vi "dfd_Get Filter Freq Resp on Freq Pts.vi"(6 "fs [Hz]":dbl, 7 "freqs [Hz]":dbl[](array[numeric]), 8 "error in (no error)":errorcluster, 10 "coef source":enum16{"Original", "Current", "Quantized"}(ring), 11 "filter in":T1 {"mSRate_QSettings"."source" items=["Coef a/k"=0, "Coef b/v"=7, "Input"=1, "Output"=2, "Multiplicand"=3, "Product"=4, "Sum"=5, "Delay"=6, "Gain"=8]}) -> (0 "error out":errorcluster, 3 "freq response":cdb[](array[numeric]))   [LabVIEW 2017, in "NI_DigFilterLicensed.lvlib"]
uses:
  <vilib>/addons/Digital Filter Design/NI_DigFilterLicensed.lvlib
  <vilib>/addons/Digital Filter Design/_Objects.llb/DFD Filter Obj.ctl
  <vilib>/addons/Digital Filter Design/_Objects.llb/DFD Filter Coef.ctl
  <vilib>/addons/Digital Filter Design/_Objects.llb/DFD Filter Structure Type Selector.ctl
  <vilib>/addons/Digital Filter Design/_Objects.llb/dfd_Internal Quantization Settings.ctl
  <vilib>/addons/Digital Filter Design/_Objects.llb/dfd_Internal Quantization Srcs.ctl
  <vilib>/addons/Digital Filter Design/_Objects.llb/DFD Coef Norm Type.ctl
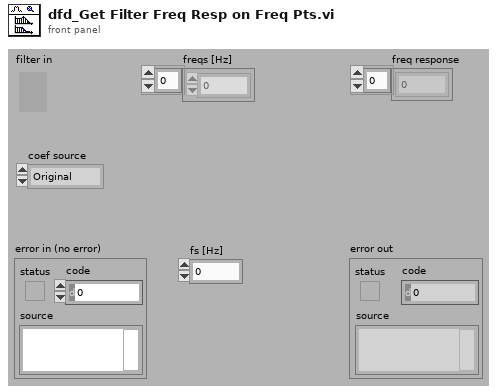
[diagram p1: front panel]
types:
  T1 = typedef "NI_DigFilterLicensed.lvlib/DFD Filter Obj.ctl" = cluster{"mSRate_Fs":dbl, "mSRate_Version":string, "mSRate_Comments":string, "mSRate_OrgCoef":T2, "mSRate_CurCoef":T2, "mSRate_Quantized?":bool, "mSRate_QCoef":T2, "mSRate_QSettings":T4[], "mSRate_Order":i32, "mSRate_Scaling":cluster{"mSRate_ScaleByPowerOf2?":bool, "mSRate_ScaleType":T6}}
  T2 = typedef "NI_DigFilterLicensed.lvlib/DFD Filter Coef.ctl" = cluster{"type":T3, "gain":dbl, "coef a (k)":dbl[], "coef b (v)":dbl[]}
  T3 = typedef "NI_DigFilterLicensed.lvlib/DFD Filter Structure Type Selector.ctl" = enum16{"Undefined", "FIR Direct Form", "FIR Direct Form Transposed", "FIR Symmetric", "FIR Antisymmetric", "IIR Direct Form I", "IIR Direct Form I Transposed", "IIR Direct Form II", "IIR Direct Form II Transposed", "IIR Cascaded Second Order Sections Form I", "IIR Cascaded Second Order Sections Form I Transposed", "IIR Cascaded Second Order Sections Form II", "IIR Cascaded Second Order Sections Form II Transposed", "Lattice Allpass (basic sections)", "Lattice Allpass (one multiplier sections)", "Lattice Allpass (normalized sections)", "Lattice AR (basic sections)", "Lattice AR (one multiplier sections)", "Lattice AR (normalized sections)", "Lattice MA (minimum phase)", "Lattice MA (maximum phase)", "Lattice ARMA (basic sections)", "Lattice ARMA (one multiplier sections)", "Lattice ARMA (normalized sections)"}
  T4 = typedef "NI_DigFilterLicensed.lvlib/dfd_Internal Quantization Settings.ctl" = cluster{"source":T5, "wl":i16, "iwl":i16, "overflow mode":enum16{"Saturation", "Wrap"}, "rounding mode":enum16{"Nearest", "Truncation"}, "signed?":bool}
  T5 = typedef "NI_DigFilterLicensed.lvlib/dfd_Internal Quantization Srcs.ctl" = u16
  T6 = typedef "NI_DigFilterLicensed.lvlib/DFD Coef Norm Type.ctl" = enum16{"No Norm", "Time Domain 1-Norm", "Time Domain 2-Norm", "Time Domain Inf-Norm"}
  T7 = typedef "NI_DigFilterLicensed.lvlib/DFD Filter Structure Id.ctl" = enum16{"Undefined", "FIR", "IIR Direct", "IIR SOS", "IIR Allpass", "IIR AR", "IIR ARMA"}
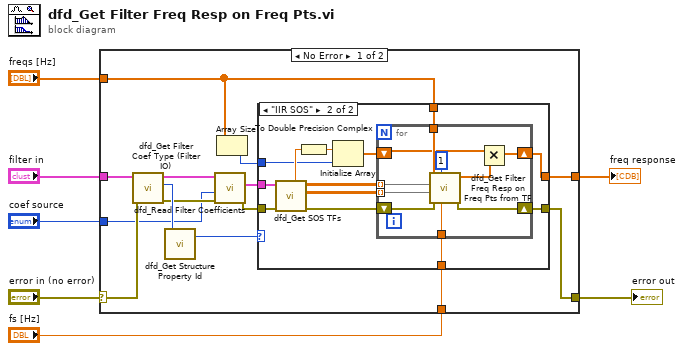
[diagram p0: block diagram]
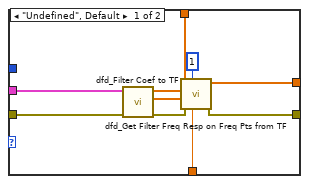
[diagram p2: hidden frame]
diagram:
  n1 = case shown="No Error" "error in (no error)" {
    selector: "error in (no error)" -> [w18 w55]
    tunnel: "coef source" -> [w14 _]
    tunnel: [w21 _] -> w6
    tunnel: "filter in" -> [w19 _]
    tunnel: "freqs [Hz]" -> [w10 _]
    tunnel: "fs [Hz]" -> [w20 _]
    tunnel: [w8 w55] -> w1
    frame No Error {
      n2 = call <vilib>:"dfd_Get Filter Coef Type (Filter IO).vi"("error in (no error)"=w18, "filter in"=w19) -> ("error out"=w15:errorcluster, "type"=w17:T3, "filter out"=w16:T1)  [unwired: 1 in, 6 out]
      n3 = call <vilib>:"dfd_Get Structure Property Id.vi"("structure type"=w17) -> ("filter structure id"=w13:T7)  [unwired: 1 out]
      n4 = call <vilib>:"dfd_Read Filter Coefficients.vi"("error in (no error)"=w15, "coef source"=w14, "filter in"=w16) -> ("error out"=w11:errorcluster, "filter coef"=w12:T2)  [unwired: 7 out]
      n5 = Array Size(array=w10) -> (size(s)=w9:i32)
      n6 = case shown="\"IIR SOS\"" w13 {
        tunnel: [w30 w37] -> w21
        tunnel: w10 -> [w26 w39]
        tunnel: w20 -> [w25 w38]
        tunnel: w12 -> [w24 w44]
        tunnel: w11 -> [w23 w43]
        tunnel: w9 -> [_ w34]
        tunnel: [w22 w32] -> w8
        frame "Undefined", Default {
          n7 = call <vilib>:"dfd_Filter Coef to TF.vi"("error out"=w23, "filter coef"=w24) -> ("error"=w29:errorcluster, "denominator"=w28:dbl[], "numerator"=w27:dbl[])  [unwired: 7 out]
          n8 = call <vilib>:"dfd_Get Filter Freq Resp on Freq Pts from TF.vi"("fs [Hz]"=w25, "factor"=1, "error in (no error)"=w29, "den"=w28, "num"=w27, "freq points [Hz]"=w26) -> ("error out"=w22:errorcluster, "freq response"=w30:cdb[])  [unwired: 4 out]
        }
        frame "IIR SOS" {
          n9 = call <vilib>:"dfd_Get SOS TFs.vi"("error in (no error)"=w43, "filter coef"=w44) -> ("error out"=w40:errorcluster, "dens"=w41:dbl[][], "nums"=w42:dbl[][], "gain"=w35:dbl)  [unwired: 6 out]
          n10 = To Double Precision Complex(1:w35) -> (0:w33:cdb)
          n11 = Initialize Array(w33, w34) -> (w36:cdb[])
          n12 = for {
            tunnel: w42 -> [w54] mode=indexing
            tunnel: w41 -> [w53] mode=indexing
            shift-right: [w49] -> w32
            shift-left: w40 -> [w50]
            tunnel: w39 -> [w52]
            tunnel: w38 -> [w51]
            shift-right: [w47] -> w37
            shift-left: w36 -> [w45]
            n13 = call <vilib>:"dfd_Get Filter Freq Resp on Freq Pts from TF.vi"("fs [Hz]"=w51, "factor"=1, "error in (no error)"=w50, "den"=w53, "num"=w54, "freq points [Hz]"=w52) -> ("error out"=w49:errorcluster, "freq response"=w46:cdb[])  [unwired: 4 out]
            n14 = Multiply(x=w45, y=w46) -> (x*y=w47:cdb[])
          }
        }
      }
    }
    frame Error {
    }
  }
  "freq response" <- w6
  "error out" <- w1
